vi "Main_menu.vi"() -> ()   [LabVIEW 2021]
doc: "The main menu function acts as the focal point for navigating and utilizing the diverse range of features and capabilities within our application. When users initiate the application, they encounter a user-friendly menu interface, offering a variety of options that cater to their specific requirements.\n Key functionalities include:\n Initiating window plots for data visualization\n Establishing communication with microcontrollers\n Implementing robust error handling mechanisms"
uses:
  <vilib>/event_ctls.llb/lveventtype.ctl
  <vilib>/Utility/file.llb/Write Delimited Spreadsheet (DBL).vi
panel:
  out "Iteration \ninterval (ms)":u32
  in  "Clear error":bool
  out "Error":bool
  out "Close":bool
  in  "?":T1(tab)
  in  "New_plot_window":bool
  in  "List of active windows":i32(listbox)
  in  "Close all plots":bool
  in  "CSV Path for Signals":path
  in  "Instant\nRefresh \ntime (ms)":i32
  out "Trace total samples":i32
  in  "Start record":bool
  in  "Continuous\nRefresh \ntime (ms)":i32
  in  "Global Mode":enum32{"Item 0", "Item 1"}(radio)
  in  "Samples per signal":u32
  in  "Trace names":string(combo)
  out "Total number signals":i32
  in  "Save CSV":bool
  in  "Stop":bool
  out "Run_record":bool
  in  "CTRL enable":bool
  in  "Save CTRL parameters":bool
  out "Total\ncontrols":i32
  in  "# Control":string(combo)
  in  "CS enable":bool
  out "CS status":i32
  in  "CS_IF_Params":T2 {"CS_Duty" min=0 max=1}
  out "Connected":bool
  out "Saved":bool
  in  "Save configuration":bool
  in  "Port":i32
  in  "Hostname":string
  in  "Timeout ms":i32
  in  "Send message":bool
  in  "Index window":i32
  in  "msj":string
  out "error out":errorcluster
  # "ctrl_if:0\nctrl: 2\nset parm: 2"
  # "In this section the user can send a message or data to a defined active window plot. \nJust to develop."
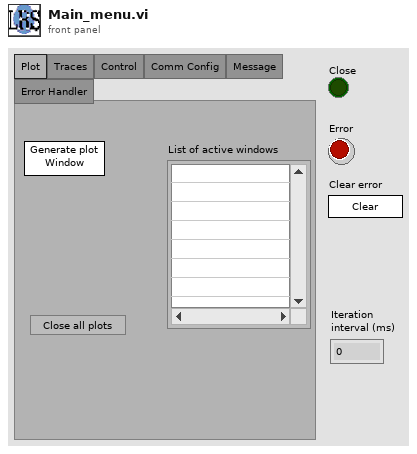
[diagram p1: front panel]
types:
  T1 = enum32{"Plot", "Traces", "Control", "Comm Config", "Message", "Error Handler"}
  T2 = cluster{"SET_PARAMETERS":i32, "CTLR":i32, "CS_Duty":sgl, "CTRL_IF_SET":i32}
  T3 = cluster{"Port":i32, "hostname":string, "status":bool, "timeout ms":i32, "TRACES_NAMES":string[], "Refresh time ms":i32, "Mode":enum32{"Item 0", "Item 1"}, "Start":bool, "DATA":sgl[][], "SIGNALS_NAMES":string[], "NB_SIGNALS":i32, "NB_TRACES":i32, "ID_TRACE":i32, "Mark":bool, "Counter":i32, "CTRLs_NAMES":string[], "NB_Ctrls":i32, "CS enable?":bool, "CS ID":i32}
  T4 = enum8{"Enabled", "Disabled", "Disabled and Grayed Out"}
  T5 = typedef "lveventtype.ctl" = enum32{"Null", "Timeout", "Annotation Menu Selection", "Annotation Menu Selection?", "App Instance Close", "App Instance Close?", "Autoscale Range Change", "Bookmark Info Change", "Cell Edit", "Cell Edit?", "Cursor Grab", "Cursor Grab?", "Cursor Menu Selection", "Cursor Menu Selection?", "Cursor Move", "Cursor Release", "Data Change", "Direction Change", "Display State Change", "Drag Ended", "Drag Enter", "Drag Leave", "Drag Over", "Drag Source Update", "Drag Starting", "Drag Starting?", "Drop", "Exec State Change", "Key Down", "Key Down?", "Key Repeat", "Key Repeat?", "Key Up", "Listbox Double Click", "Menu Activation?", "Menu Selection (App)", "Menu Selection? (App)", "Menu Selection (User)", "Mouse Down", "Mouse Down?", "Mouse Enter", "Mouse Leave", "Mouse Move", "Mouse Up", "Mouse Wheel", "NI Security User Change (App)", "Pane Size", "Panel Close", "Panel Close?", "Panel Resize", "Plot Attribute Change", "Scale Range Change", "Shortcut Menu Activation?", "Shortcut Menu Selection (App)", "Shortcut Menu Selection? (App)", "Shortcut Menu Selection (User)", "Tree Double Click", "Tree Drag", "Tree Drag?", "Tree Drop", "Tree Drop?", "Tree Item Close", "Tree Item Close?", "Tree Item Open", "Tree Item Open?", "User Event", "Value Change"}
  T6 = enum16{"open", "replace", "create", "open or create", "replace or create", "replace or create with confirmation"}
  T7 = enum32{"Invalid", "Standard", "Closed", "Hidden", "Minimized", "Maximized"}
  T8 = enum32{"invalid app kind", "Development System", "Run Time System", "Student Edition", "Embedded LabVIEW", "Evaluation", "Custom"}
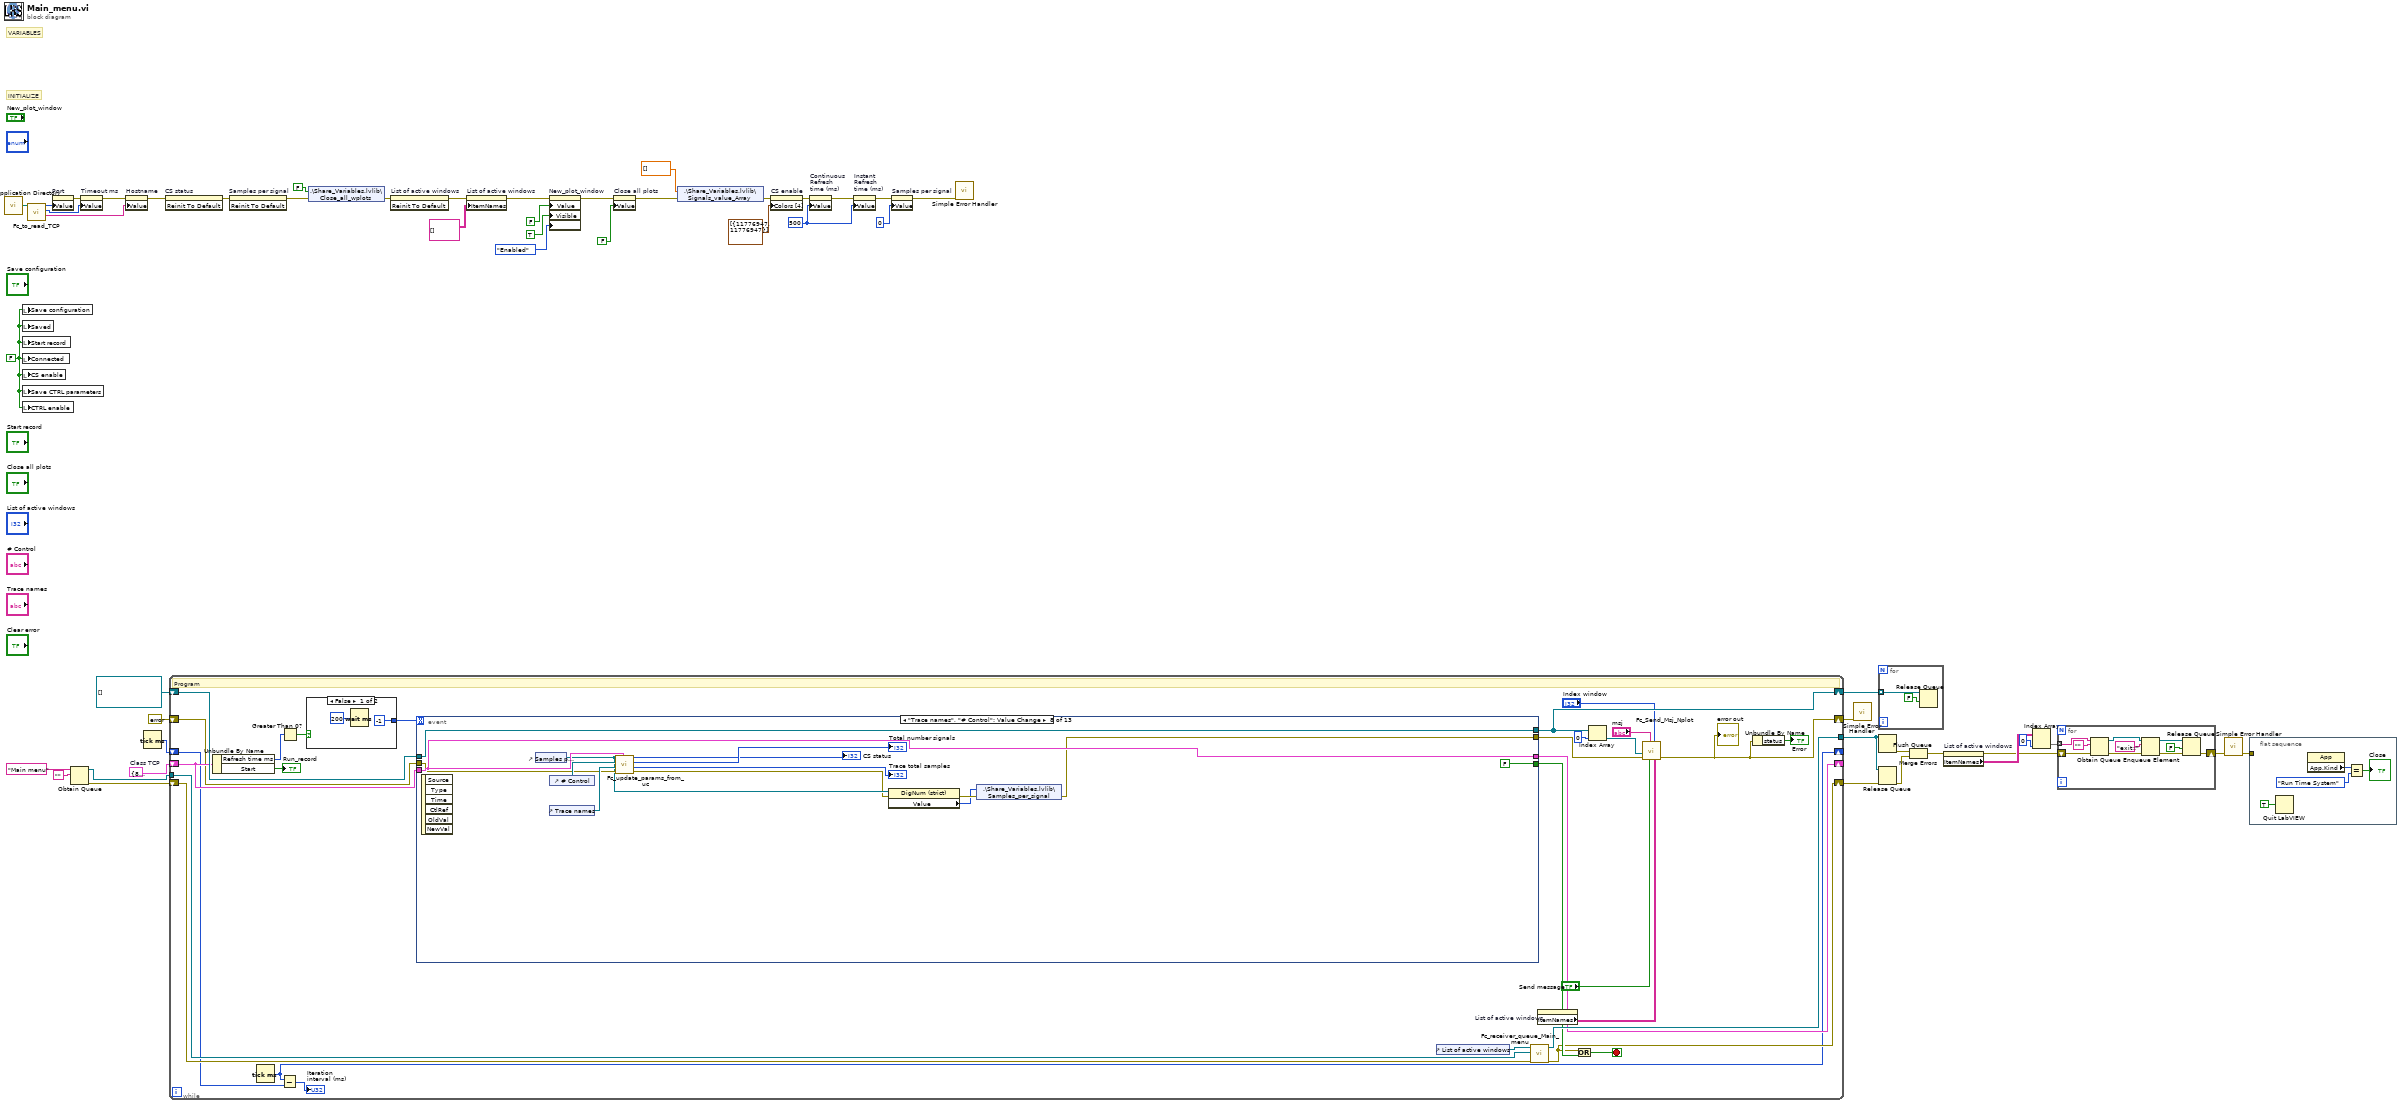
[diagram p0: block diagram]
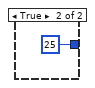
[diagram p2: hidden frame]
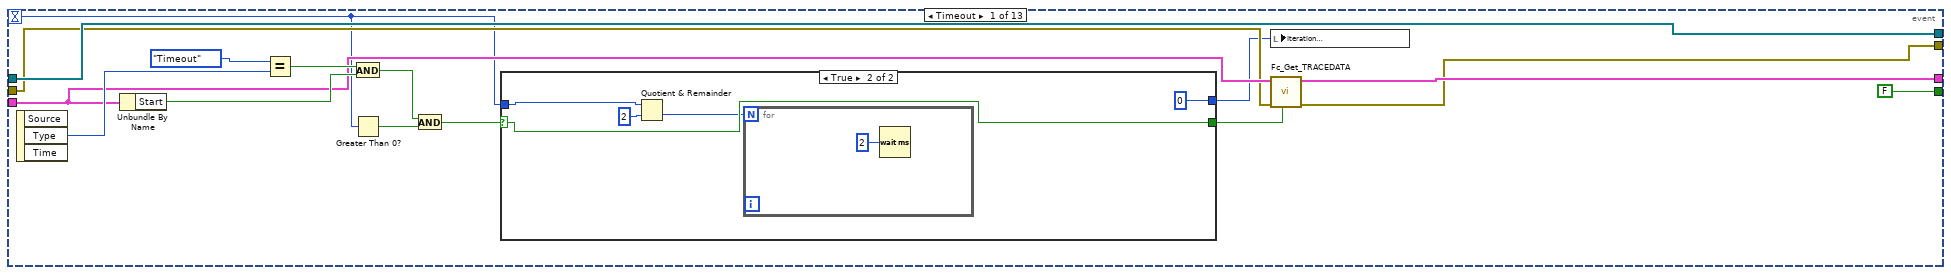
[diagram p3: hidden frame]
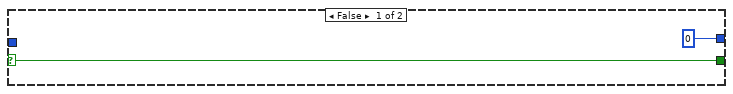
[diagram p4: hidden frame]
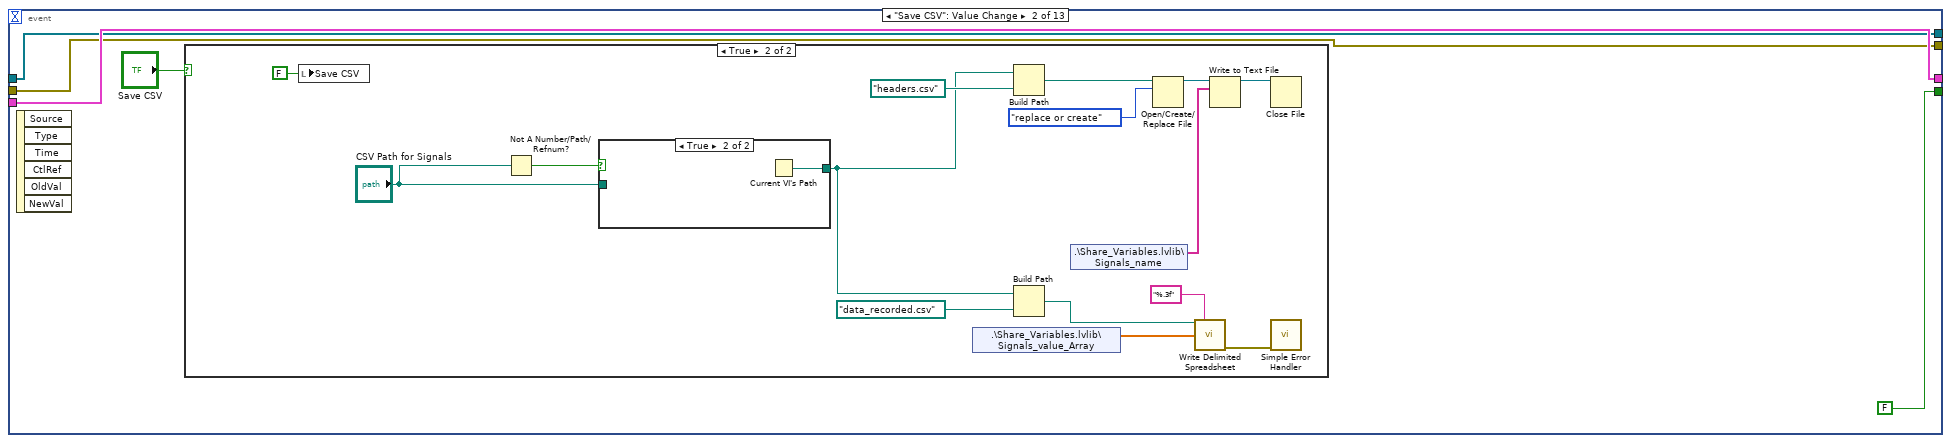
[diagram p5: hidden frame]
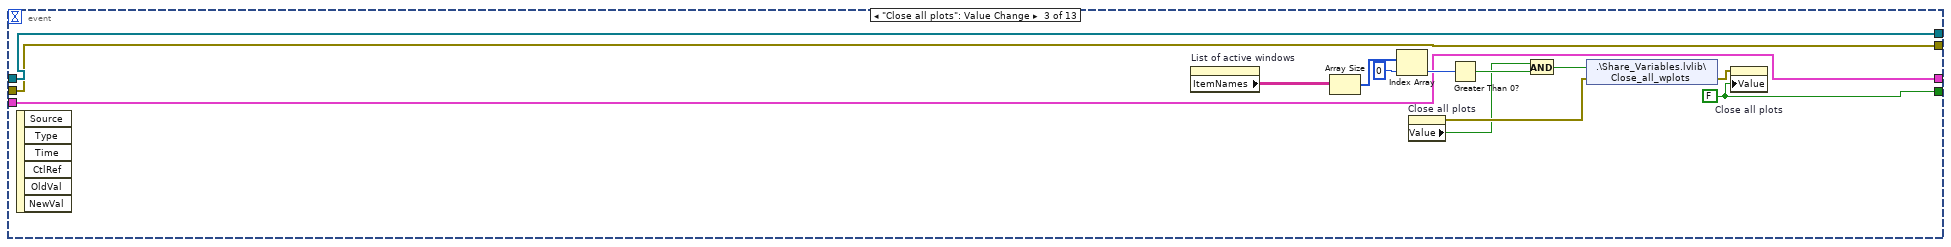
[diagram p8: hidden frame]
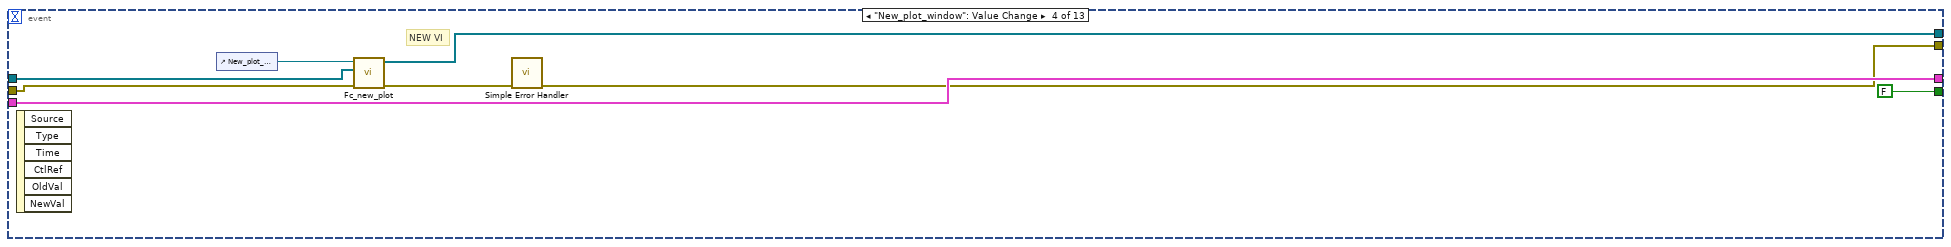
[diagram p9: hidden frame]
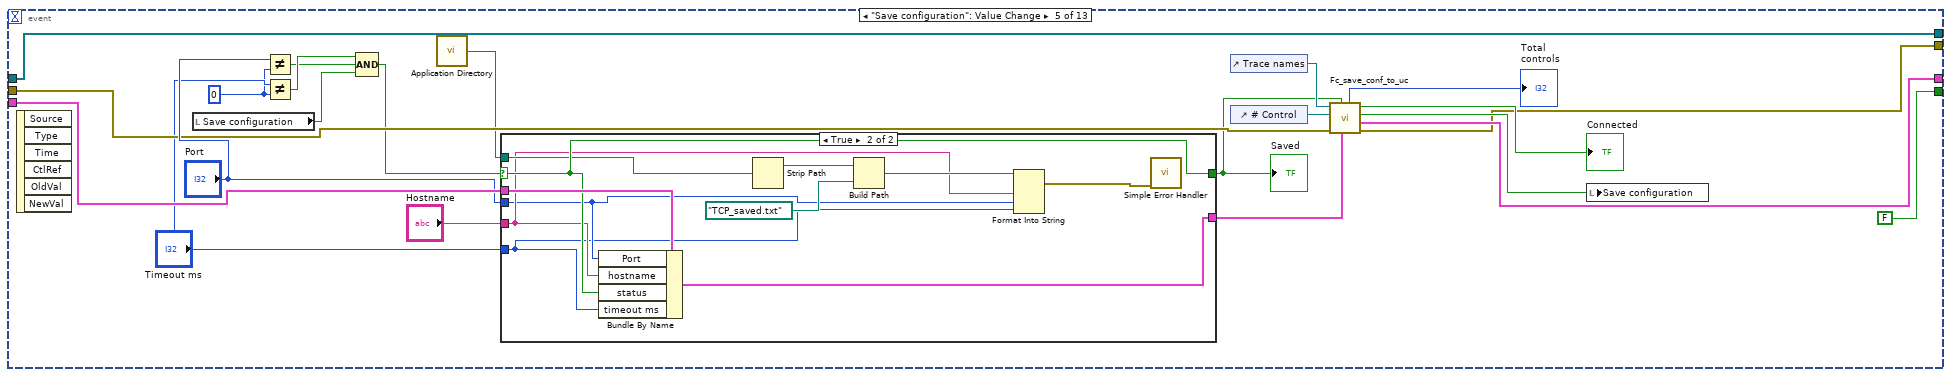
[diagram p10: hidden frame]
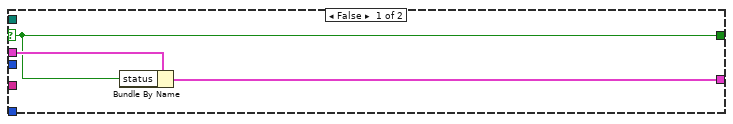
[diagram p11: hidden frame]
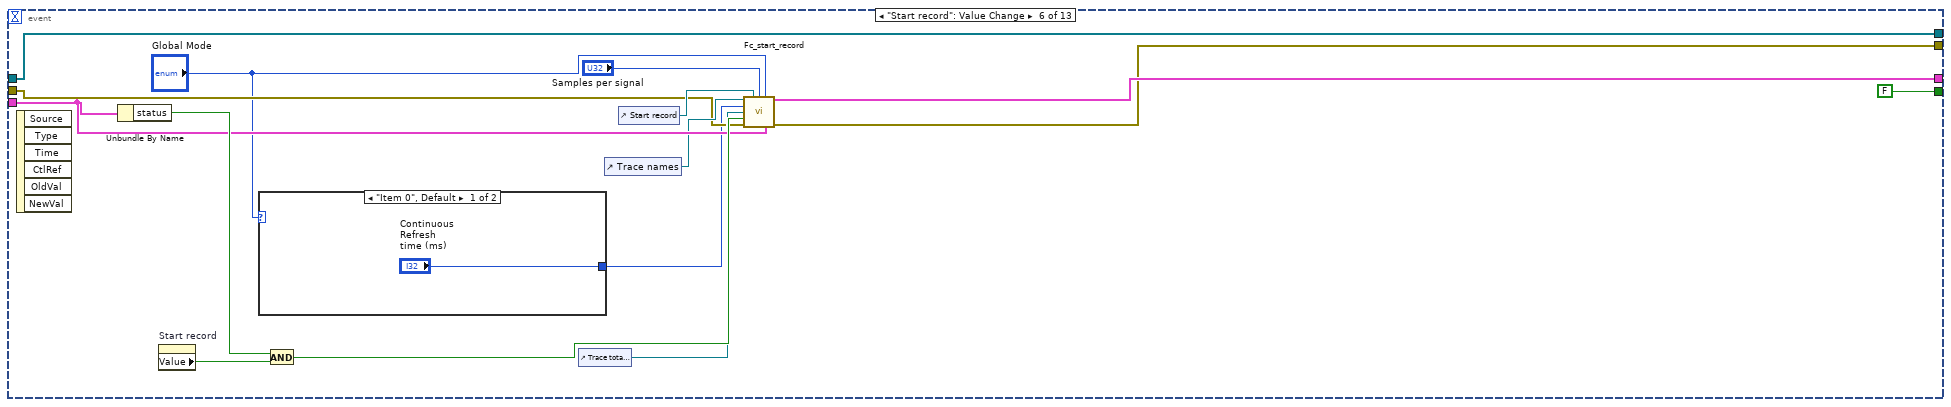
[diagram p12: hidden frame]
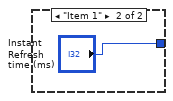
[diagram p13: hidden frame]
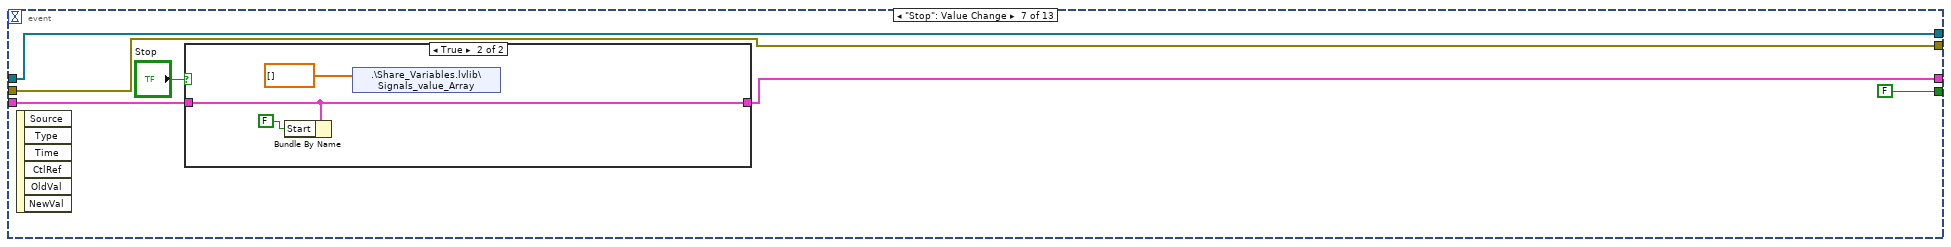
[diagram p14: hidden frame]
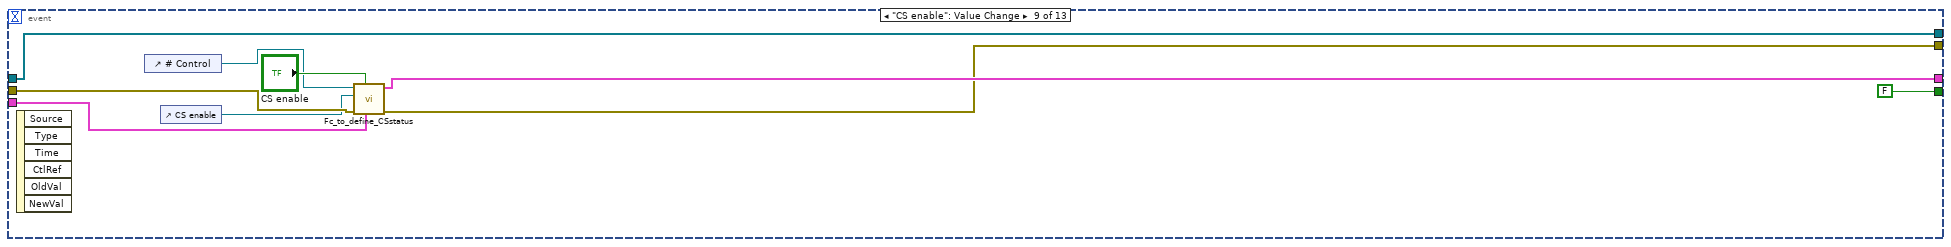
[diagram p16: hidden frame]
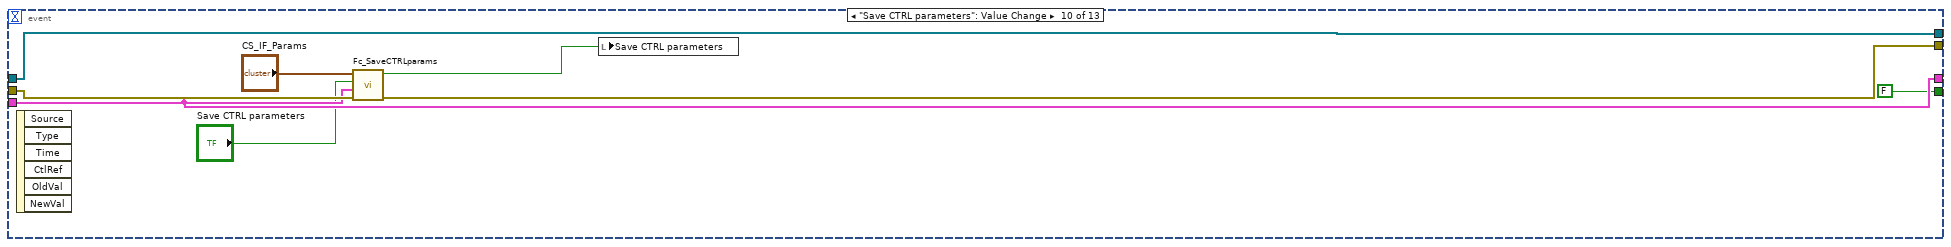
[diagram p17: hidden frame]
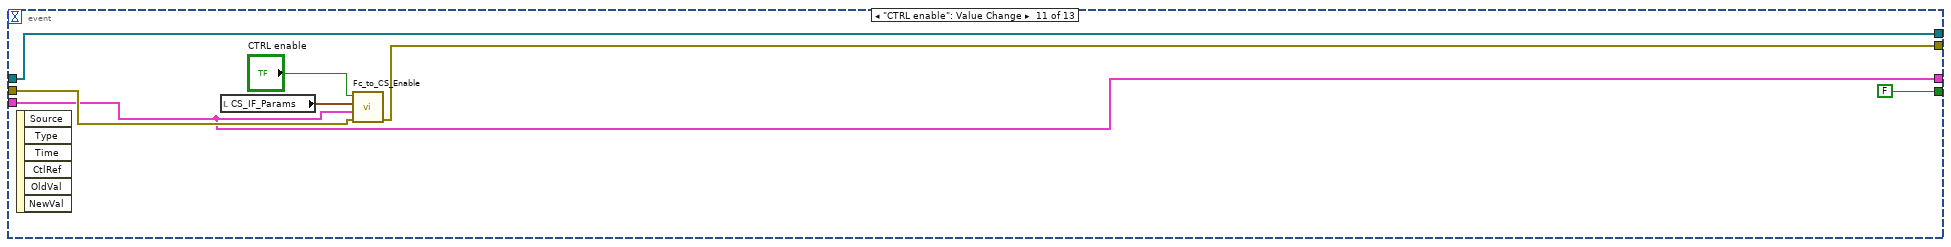
[diagram p18: hidden frame]
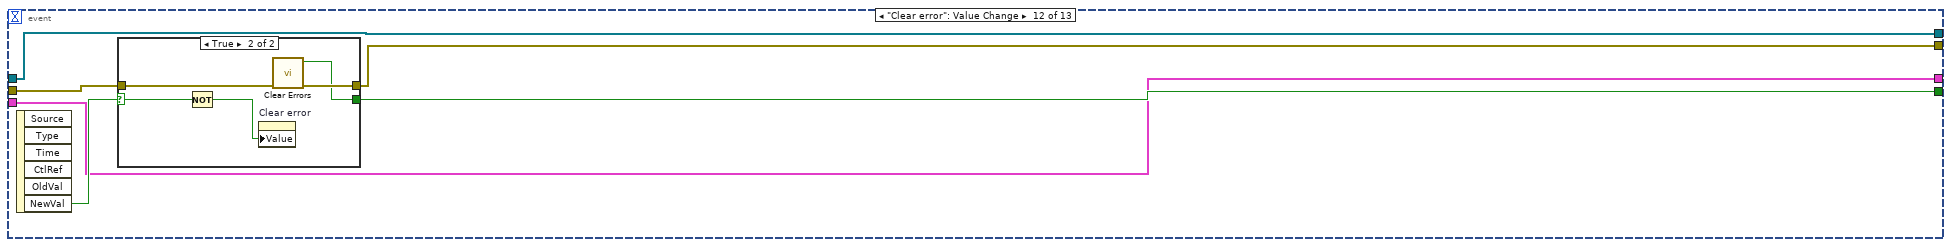
[diagram p19: hidden frame]
diagram:
  w9 = 500 ("Refresh \ntime (ms)")
  w32 = T3 {"Port"=8085, "hostname"="", "status"=FALSE, "timeout ms"=1000, "TRACES_NAMES"=[], "Refresh time ms"=-1, "Mode"=enum."Item 0", "Start"=FALSE, "DATA"=[], "SIGNALS_NAMES"=[], "NB_SIGNALS"=0, "NB_TRACES"=0, "ID_TRACE"=0, "Mark"=FALSE, "Counter"=0, "CTRLs_NAMES"=[], "NB_Ctrls"=0, "CS enable?"=FALSE, "CS ID"=0}  # Class TCP
  w21 = FALSE ("Save conf")
  # "INITIALIZE"
  # "VARIABLES"
  n1 = call <vilib>:"Application Directory.vi"() -> ("Application Directory"=w2:path)
  n2 = local write "Save configuration"(w21) -> ()
  n3 = local write "Saved"(w21) -> ()
  n4 = local write "Start record"(w21) -> ()
  n5 = local write "Connected"(w21) -> ()
  n6 = local write "CS enable"(w21) -> ()
  n7 = local write "Save CTRL parameters"(w21) -> ()
  n8 = local write "CTRL enable"(w21) -> ()
  n9 = call "Fc_to_read_TCP.vi"("path_mainmenu"=w2) -> ("Hhostname"=w5:string, "Timeout ms"=w3:i32, "Port"=w4:i32)  [unwired: 8 in]
  n10 = property on="Port" class="DigNum (strict)"("Value"=w4) -> (error out=w31:errorcluster)  [unwired: 2 in, 1 out]
  n11 = Obtain Queue(name (unnamed)="Main menu", element data type="") -> (queue out=w44:refnum<queue>, error out=w42:errorcluster)  [unwired: 3 in, 1 out]
  n12 = property on="Timeout ms" class="DigNum (strict)"(error in=w31, "Value"=w3) -> (error out=w27:errorcluster)  [unwired: 1 in, 1 out]
  n13 = property on="Hostname" class="Str"(error in=w27, "Value"=w5) -> (error out=w17:errorcluster)  [unwired: 1 in, 1 out]
  n14 = Tick Count (ms)() -> (millisecond timer value=w1:u32)
  n15 = invoke on="CS status" class="DigNum (strict)" method="Reinit To Default"(error in=w17) -> (error out=w26:errorcluster)  [unwired: 2 in, 2 out]
  n16 = while {
    shift-right: [w70] -> w48
    shift-left: refnum<queue>[] [] -> [w79]
    tunnel: w44 -> [w78]
    tunnel: [w77] -> w35
    shift-right: [w59] -> w43
    shift-left: w42 -> [w76]
    shift-right: [w75] -> _
    shift-left: w32 -> [w74]
    shift-right: [w64] -> w14
    shift-left: errorcluster {"status"=FALSE, "code"=0, "source"=""} ("error out") -> [w65]
    shift-right: [w52] -> _
    shift-left: w1 -> [w53]
    stop <- w60 stop-if-true
    # "Program"
    n17 = Unbundle By Name(w74) -> ("Refresh time ms"=w56:i32, "Start"=→"Run_record":bool)
    n18 = Tick Count (ms)() -> (millisecond timer value=w52:u32)
    n19 = Subtract(x=w52, y=w53) -> (x-y=→"Iteration \ninterval (ms)":u32)
    n20 = Greater Than 0?(x=w56) -> (x > 0?=w57:bool)
    n21 = case shown="False" w57 {
      tunnel: [-1 25] -> w55
      frame False {
        n22 = Wait (ms)(milliseconds to wait=u32 200) -> ()  [unwired: 1 out]
      }
      frame True {
      }
    }
    n23 = event shown="[7] \"Trace names\", \"# Control\": Value Change" {
      selector: _ -> [_ _ _ _ _ _ _ _ _ _ _ _ _]
      dyn-events: _ -> [_ _ _ _ _ _ _ _ _ _ _ _ _]
      timeout: w55 -> [w85 _ _ _ _ _ _ _ _ _ _ _ _]
      tunnel: [FALSE ("f") FALSE ("specific error cleared?") w132 FALSE ("f") FALSE ("f") FALSE ("f") FALSE ("specific error cleared?") FALSE ("f") FALSE ("specific error cleared?") FALSE ("specific error cleared?") FALSE ("specific error cleared?") w253 w270] -> w61
      tunnel: [w98 w108 w141 w149 w152 w187 w204 w218 w228 w237 w245 w251 w269] -> w70
      tunnel: w79 -> [w98 w108 w141 w148 w152 w187 w204 w218 w228 w237 w245 w251 w269]
      tunnel: [w92 w110 w136 w146 w165 w197 w206 w225 w235 w242 w249 w252 w264] -> w75
      tunnel: w74 -> [w93 w110 w136 w146 w171 w198 w207 w225 w234 w242 w249 w252 w264]
      tunnel: w65 -> [w90 w109 w135 w144 w168 w191 w205 w219 w231 w243 w250 w255 w268]
      tunnel: [w89 w109 w135 w142 w153 w190 w205 w213 w229 w238 w246 w254 w268] -> w62
      event Timeout {
        n24 = event-data() -> ("Type"=w96:T5)  [unwired: 1 in, 2 out]
        n25 = Unbundle By Name(w93) -> ("Start"=w94:bool)
        n26 = Equal?(x=lveventtype."Timeout" ("Type"), y=w96) -> (x = y?=w95:bool)
        n27 = And(x=w95, y=w94) -> (x .and. y?=w88:bool)
        n28 = Greater Than 0?(x=w85) -> (x > 0?=w87:bool)
        n29 = And(x=w88, y=w87) -> (x .and. y?=w86:bool)
        n30 = case shown="True" w86 {
          selector: w86 -> [w100 w105]
          tunnel: w85 -> [_ w104]
          tunnel: [w100 w105] -> w84
          tunnel: [0 ("counter (2ms)") 0 ("counter (2ms)")] -> w83
          frame False {
          }
          frame True {
            n31 = Quotient & Remainder(x=w104, y=2) -> (floor(x/y)=w102:i32)  [unwired: 1 out]
            n32 = for {
              N: w102 -> [_]
              n33 = Wait (ms)(milliseconds to wait=u32 2) -> ()  [unwired: 1 out]
            }
          }
        }
        n34 = local write "Iteration \ninterval (ms)"(w83) -> ()
        n35 = call "Fc_Get_TRACEDATA.vi"("Start+timeout?"=w84, "error in (no error)"=w90, "Class TCP in"=w93) -> ("error out"=w89:errorcluster, "Class TCP out"=w92:T3)  [unwired: 7 in]
      }
      event "Save CSV": Value Change {
        n36 = event-data() -> ()  [unwired: 1 in, 6 out]
        n37 = case shown="True" "Save CSV" {
          frame False {
          }
          frame True {
            n38 = local write "Save CSV"(FALSE ("CSV")) -> ()
            n39 = Not A Number/Path/Refnum?(number/path/refnum="CSV Path for Signals") -> (NaN/Path/Refnum?=w114:bool)
            n40 = case shown="True" w114 {
              tunnel: [w127 w128] -> w113
              tunnel: "CSV Path for Signals" -> [w127 _]
              frame False {
              }
              frame True {
                n41 = Current VI's Path() -> (path=w128:path)
              }
            }
            n42 = shared-variable ".\\Share_Variables.lvlib\\Signals_value_Array"() -> (w123:dbl[])  [unwired: 1 in, 1 out]
            n43 = Build Path(base path=w113, name or relative path=path "headers.csv") -> (appended path=w120:path)
            n44 = Build Path(base path=w113, name or relative path=path "data_recorded.csv") -> (appended path=w122:path)
            n45 = shared-variable ".\\Share_Variables.lvlib\\Signals_name"() -> (w117:string[])  [unwired: 1 in, 1 out]
            n46 = Open/Create/Replace File(file path (use dialog)=w120, operation (0:open)=T6."replace or create") -> (refnum out=w118:refnum<file>)  [unwired: 4 in, 2 out]
            n47 = call-poly <vilib>:"Write Delimited Spreadsheet.vi"("file path (dialog if empty)"=w122, "format (%.3f)"="%.3f", "1D data"=w123) -> ("error out"=w124:errorcluster)  [unwired: 11 in, 1 out]
            n48 = Write to Text File(file (use dialog)=w118, text=w117) -> (refnum out=w116:refnum<file>)  [unwired: 2 in, 2 out]
            n49 = Close File(refnum=w116) -> ()  [unwired: 1 in, 2 out]
            n50 = call <vilib>:"Simple Error Handler.vi"("error in (no error)"=w124) -> ()  [unwired: 4 in, 5 out]
          }
        }
      }
      event "Close all plots": Value Change {
        w132 = FALSE ("f")
        n51 = event-data() -> ()  [unwired: 1 in, 6 out]
        n52 = property on="List of active windows" class="MCListbox (strict)"() -> ("ItemNames"=w137:string[][])  [unwired: 2 in, 2 out]
        n53 = Array Size(array=w137) -> (size(s)=w140:i32[])
        n54 = Index Array(array=w140, index=0) -> (element=w138:i32)
        n55 = property on="Close all plots" class="Bool (strict)"() -> (error out=w130:errorcluster, "Value"=w129:bool)  [unwired: 2 in, 1 out]
        n56 = Greater Than 0?(x=w138) -> (x > 0?=w131:bool)
        n57 = And(x=w129, y=w131) -> (x .and. y?=w134:bool)
        n58 = shared-variable ".\\Share_Variables.lvlib\\Close_all_wplots"(w134, error in=w130) -> (error out=w133:errorcluster)
        n59 = property on="Close all plots" class="Bool (strict)"(error in=w133, "Value"=w132) -> ()  [unwired: 1 in, 2 out]
      }
      event "New_plot_window": Value Change {
        # "NEW VI"
        n60 = event-data() -> ()  [unwired: 1 in, 6 out]
        n61 = control-ref of="New_plot_window"() -> (w145:refnum<vi>)
        n62 = call "Fc_new_plot.vi"("error in (no error)"=w144, "Array in"=w148, "Boolean in"=w145) -> ("error out"=w143:errorcluster, "Array out"=w149:refnum<queue>[])  [unwired: 7 in]
        n63 = call <vilib>:"Simple Error Handler.vi"("error in (no error)"=w143) -> ("error out"=w142:errorcluster)  [unwired: 4 in, 4 out]
      }
      event "Save configuration": Value Change {
        w154 = 0 ("y")
        n64 = event-data() -> ()  [unwired: 1 in, 6 out]
        n65 = local read "Save configuration"() -> (w156:bool)
        n66 = Not Equal?(x="Port", y=w154) -> (x != y?=w157:bool)
        n67 = Not Equal?(x="Timeout ms", y=w154) -> (x != y?=w158:bool)
        n68 = Compound Arithmetic op=AND(w158, w157, w156) -> (w155:bool)
        n69 = call <vilib>:"Application Directory.vi"() -> ("Application Directory"=w150:path)
        n70 = case shown="True" w155 {
          selector: w155 -> [w172 w183]
          tunnel: [w172 w183] -> w151
          tunnel: "Port" -> [_ w177]
          tunnel: "Hostname" -> [_ w178]
          tunnel: [w174 w184] -> w166
          tunnel: w171 -> [w173 w185]
          tunnel: "Timeout ms" -> [_ w176]
          tunnel: w150 -> [_ w179]
          frame False {
            n71 = Bundle By Name(cluster=w173, "status"=w172) -> (w174:T3)
          }
          frame True {
            n72 = Bundle By Name(cluster=w185, "Port"=w177, "hostname"=w178, "status"=w183, "timeout ms"=w176) -> (w184:T3)
            n73 = Strip Path(path=w179) -> (stripped path=w182:path)  [unwired: 1 out]
            n74 = Build Path(base path=w182, name or relative path=path "TCP_saved.txt" ("default name")) -> (appended path=w180:path)
            n75 = Format Into String(initial string=w180, w178, w177, w176) -> (error out=w175:errorcluster)  [unwired: 2 in, 1 out]
            n76 = call <vilib>:"Simple Error Handler.vi"("error in (no error)"=w175) -> ()  [unwired: 4 in, 5 out]
          }
        }
        "Saved" <- w151
        n77 = control-ref of="Trace names"() -> (w160:refnum<vi>)
        n78 = control-ref of="# Control"() -> (w159:refnum<vi>)
        n79 = call "Fc_save_conf_to_uc.vi"("Class TCP in"=w166, "Saved configuration?"=w151, "error in (no error)"=w168, "CmbBox Refnum in"=w159, "ComboBox in"=w160) -> ("error out"=w153:errorcluster, "Class TCP out"=w165:T3, "Save conf?"=w167:bool, "Connected?"=→"Connected":bool, "NB_CSs"=→"Total\ncontrols":i32)  [unwired: 2 in]
        n80 = local write "Save configuration"(w167) -> ()
      }
      event "Start record": Value Change {
        n81 = event-data() -> ()  [unwired: 1 in, 6 out]
        n82 = Unbundle By Name(w198) -> ("status"=w200:bool)
        n83 = property on="Start record" class="Bool (strict)"() -> ("Value"=w195:bool)  [unwired: 2 in, 2 out]
        n84 = case shown="\"Item 0\", Default" "Global Mode" {
          tunnel: ["Continuous\nRefresh \ntime (ms)" "Instant\nRefresh \ntime (ms)"] -> w188
          frame "Item 0", Default {
          }
          frame "Item 1" {
          }
        }
        n85 = And(x=w200, y=w195) -> (x .and. y?=w199:bool)
        n86 = control-ref of="Trace total samples"() -> (w192:refnum<vi>)
        n87 = control-ref of="Trace names"() -> (w194:refnum<vi>)
        n88 = control-ref of="Start record"() -> (w193:refnum<vi>)
        n89 = call "Fc_start_record.vi"("Trace names"=w194, "Start record?"=w193, "Samples X Signal"="Samples per signal", "Global Mode"="Global Mode", "Refresh \ntime (ms)"=w188, "total samples?"=w192, "status+start record"=w199, "error in (no error)"=w191, "Class TCP in"=w198) -> ("Class TCP out"=w197:T3, "error out"=w190:errorcluster)  [unwired: 5 in]
      }
      event "Stop": Value Change {
        n90 = event-data() -> ()  [unwired: 1 in, 6 out]
        n91 = case shown="True" "Stop" {
          tunnel: w207 -> [w209 w211]
          tunnel: [w209 w211] -> w206
          frame False {
          }
          frame True {
            n92 = Bundle By Name(cluster=w211, "Start"=FALSE) -> ()  [unwired: 1 out]
            n93 = shared-variable ".\\Share_Variables.lvlib\\Signals_value_Array"(dbl[] [] ("Signals_value_Array")) -> ()  [unwired: 1 in, 1 out]
          }
        }
      }
      event "Trace names", "# Control": Value Change {
        n94 = event-data() -> ()  [unwired: 1 in, 6 out]
        n95 = control-ref of="Samples per signal"() -> (w217:refnum<vi>)
        n96 = control-ref of="# Control"() -> (w221:refnum<vi>)
        n97 = control-ref of="Trace names"() -> (w220:refnum<vi>)
        n98 = call "Fc_update_params_from_uc.vi"("Class TCP"=w225, "error in (no error)"=w219, "Trace names"=w220, "# Control"=w221, "SamplesPerSignal?"=w217) -> ("error out"=w214:errorcluster, "TRACE_SIZE"=→"Trace total samples":i32, "NB_TRACED_SIGNALS"=→"Total number signals":i32, "CS STATUS"=→"CS status":i32)  [unwired: 3 in]
        n99 = property class="DigNum (strict)"(reference=w217, error in=w214) -> (error out=w216:errorcluster, "Value"=w215:u32)  [unwired: 1 out]
        n100 = shared-variable ".\\Share_Variables.lvlib\\Samples_per_signal"(w215, error in=w216) -> (error out=w213:errorcluster)
      }
      event "CS enable": Value Change {
        n101 = event-data() -> ()  [unwired: 1 in, 6 out]
        n102 = control-ref of="# Control"() -> (w232:refnum<vi>)
        n103 = control-ref of="CS enable"() -> (w230:refnum<vi>)
        n104 = call "Fc_to_define_CSstatus.vi"("Class TCP in"=w234, 7:"CS enable"="CS enable", "error in (no error)"=w231, 10:"CS enable"=w230, "# Control?"=w232) -> ("error out"=w229:errorcluster, "Class TCP out"=w235:T3)  [unwired: 5 in]
      }
      event "Save CTRL parameters": Value Change {
        n105 = event-data() -> ()  [unwired: 1 in, 6 out]
        n106 = call "Fc_SaveCTRLparams.vi"("error in (no error)"=w243, "Class TCP"=w242, "Save CTRL params"="Save CTRL parameters", "CS_IF_Params"="CS_IF_Params") -> ("error out"=w238:errorcluster, "Saved CTRL params ?"=w239:bool)  [unwired: 6 in]
        n107 = local write "Save CTRL parameters"(w239) -> ()
      }
      event "CTRL enable": Value Change {
        n108 = event-data() -> ()  [unwired: 1 in, 6 out]
        n109 = local read "CS_IF_Params"() -> (w247:T2)
        n110 = call "Fc_to_CS_Enable.vi"("error in (no error)"=w250, "Class TCP"=w249, "CS_IF_Params"=w247, "CTRL enable"="CTRL enable") -> ("error out"=w246:errorcluster)  [unwired: 7 in]
      }
      event "Clear error": Value Change {
        n111 = event-data() -> ("NewVal"=w256:bool)  [unwired: 1 in, 5 out]
        n112 = case shown="True" w256 {
          selector: w256 -> [w257 w261]
          tunnel: w255 -> [w258 w263]
          tunnel: [w258 w262] -> w254
          tunnel: [w257 w259] -> w253
          frame False {
          }
          frame True {
            n113 = Not(x=w261) -> (.not. x?=w260:bool)
            n114 = property on="Clear error" class="Bool (strict)"("Value"=w260) -> ()  [unwired: 2 in, 2 out]
            n115 = call <vilib>:"Clear Errors.vi"("error in (no error)"=w263) -> ("error out"=w262:errorcluster, "specific error cleared?"=w259:bool)  [unwired: 5 in]
          }
        }
      }
      event Panel Close {
        n116 = event-data() -> ()  [unwired: 1 in, 4 out]
        n117 = control-ref of="This VI"() -> (w267:refnum<vi>)
        n118 = property class="VI"(reference=w267, "FP.State"=T7."Closed" ("Front Panel Window:State")) -> (reference out=w266:refnum<vi>)  [unwired: 1 in, 1 out]
        n119 = property class="VI"(reference=w266) -> ("FP.State"=w272:T7)  [unwired: 1 in, 2 out]
        n120 = Equal?(x=w272, y=T7."Closed") -> (x = y?=w270:bool)
      }
    }
    n121 = control-ref of="List of active windows"() -> (w68:refnum<vi>)
    n122 = call "Fc_receiver_queue_Main_menu.vi"("error in (no error)"=w76, "Queue in"=w78, "MulticolumnListbox in"=w68) -> ("error out"=w59:errorcluster, "Queue out"=w77:refnum<queue>)  [unwired: 7 in]
    n123 = property on="List of active windows" class="MCListbox (strict)"() -> ("ItemNames"=w72:string[][])  [unwired: 2 in, 2 out]
    n124 = Or(x=w59, y=w61) -> (x .or. y?=w60:bool)
    n125 = Index Array(array=w70, index=0) -> (element=w69:refnum<queue>)
    n126 = call "Fc_Send_Msj_Nplot.vi"("ItemNames"=w72, "Process in"="Index window", "Send message"="Send message", "msj"="msj", "error in (no error)"=w62, "queue in"=w69) -> ("error out"=w64:errorcluster)  [unwired: 5 in]
    "error out" <- w64
    n127 = Unbundle By Name(w64) -> ("status"=→"Error":bool)
  }
  n128 = invoke on="Samples per signal" class="DigNum (strict)" method="Reinit To Default"(error in=w26) -> (error out=w25:errorcluster)  [unwired: 2 in, 2 out]
  n129 = shared-variable ".\\Share_Variables.lvlib\\Close_all_wplots"(FALSE ("Close_all_wplots"), error in=w25) -> (error out=w30:errorcluster)
  n130 = invoke on="List of active windows" class="MCListbox (strict)" method="Reinit To Default"(error in=w30) -> (error out=w33:errorcluster)  [unwired: 2 in, 2 out]
  n131 = property on="List of active windows" class="MCListbox (strict)"(error in=w33, "ItemNames"=string[][] [] ("Item Names")) -> (error out=w24:errorcluster)  [unwired: 1 in, 1 out]
  n132 = property on="New_plot_window" class="Bool (strict)"(error in=w24, "Value"=FALSE ("New plot"), "Visible"=TRUE, "DisabledEnum"=T4."Enabled" ("Disabled")) -> (error out=w23:errorcluster)  [unwired: 1 in, 1 out]
  n133 = property on="Close all plots" class="Bool (strict)"(error in=w23, "Value"=FALSE ("Cancel Button")) -> (error out=w16:errorcluster)  [unwired: 1 in, 1 out]
  n134 = shared-variable ".\\Share_Variables.lvlib\\Signals_value_Array"(dbl[] [] ("Signals_value_Array"), error in=w16) -> (error out=w20:errorcluster)
  n135 = property on="CS enable" class="Bool (strict)"(error in=w20, "Colors [4]"=cluster{u32, u32}[] [{11776947, 11776947}]) -> (error out=w18:errorcluster)  [unwired: 1 in, 1 out]
  n136 = property on="Continuous\nRefresh \ntime (ms)" class="DigNum (strict)"(error in=w18, "Value"=w9) -> (error out=w10:errorcluster)  [unwired: 1 in, 1 out]
  n137 = property on="Instant\nRefresh \ntime (ms)" class="DigNum (strict)"(error in=w10, "Value"=w9) -> (error out=w8:errorcluster)  [unwired: 1 in, 1 out]
  n138 = property on="Samples per signal" class="DigNum (strict)"(error in=w8, "Value"=u32 0 ("Samples per signal")) -> (error out=w7:errorcluster)  [unwired: 1 in, 1 out]
  n139 = call <vilib>:"Simple Error Handler.vi"("error in (no error)"=w7) -> ()  [unwired: 4 in, 5 out]
  n140 = call <vilib>:"Simple Error Handler.vi"("error in (no error)"=w14) -> ()  [unwired: 4 in, 5 out]
  n141 = for {
    tunnel: w48 -> [w274] mode=indexing
    n142 = Release Queue(queue=w274, force destroy? (F)=FALSE) -> ()  [unwired: 1 in, 3 out]
  }
  n143 = Flush Queue(queue=w35) -> (error out=w13:errorcluster)  [unwired: 1 in, 2 out]
  n144 = Release Queue(queue=w35, error in (no error)=w43) -> (error out=w12:errorcluster)  [unwired: 1 in, 2 out]
  n145 = Merge Errors(w13, w12) -> (w11:errorcluster)
  n146 = property on="List of active windows" class="MCListbox (strict)"(error in=w11) -> (error out=w38:errorcluster, "ItemNames"=w41:string[][])  [unwired: 1 in, 1 out]
  n147 = Index Array(array=w41, index (col)=0 ("disabled index (col)")) -> (element=w39:string[])  [unwired: 1 in]
  n148 = for {
    tunnel: w39 -> [w284] mode=indexing
    shift-right: [w281] -> w37
    shift-left: w38 -> [w283]
    n149 = Obtain Queue(name (unnamed)=w284, element data type="", error in (no error)=w283) -> (queue out=w276:refnum<queue>, error out=w278:errorcluster)  [unwired: 2 in, 1 out]
    n150 = Enqueue Element(queue=w276, element="exit::", error in (no error)=w278) -> (queue out=w275:refnum<queue>, error out=w277:errorcluster)  [unwired: 1 in, 1 out]
    n151 = Release Queue(queue=w275, force destroy? (F)=FALSE, error in (no error)=w277) -> (error out=w281:errorcluster)  [unwired: 2 out]
  }
  n152 = call <vilib>:"Simple Error Handler.vi"("error in (no error)"=w37) -> ("error out"=w36:errorcluster)  [unwired: 4 in, 4 out]
  n153 = flat-sequence {
    tunnel: w36 -> [_]
    frame #0 {
      n154 = Quit LabVIEW(quit? (T)=TRUE) -> ()
      n155 = property class="App"() -> ("App.Kind"=w288:T8)  [unwired: 2 in, 2 out]
      n156 = Equal?(x=w288, y=T8."Run Time System" ("Application:Kind")) -> (x = y?=→"Close":bool)
    }
  }
